vi "API Handle Value Change - Add to Owner.vi"(8 "Error In":errorcluster, 11 "Add to Owner New Value":bool) -> (0 "Error Out":errorcluster)   [LabVIEW 2022 SP3]
doc: "Enqueues a command."
uses:
  Command.ctl
panel:
  # "Development\ncontrols/indicators useful for development and testing, but which are not outputs of the VI"
  # "Input\nInputs to the VI"
  # "Output\nOutputs of the VI"
  # "Description\n\nBlank VI with error handling case. \n\nSummarize the use of this VI in this space."
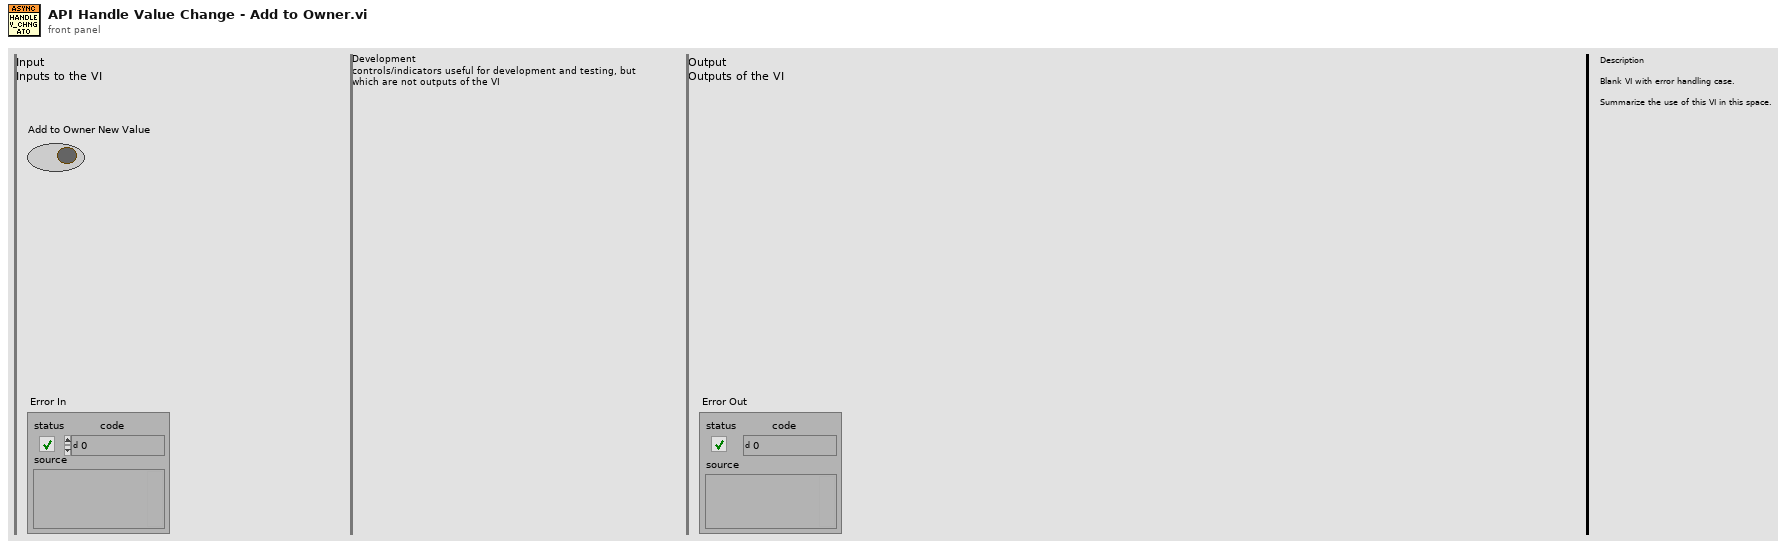
[diagram p1: front panel]
types:
  T1 = typedef "Command.ctl" = enum16{"Init Module", "Shutdown Module", "Local Error Handler", "Init Tickboxes", "Handle Value Change - Add to Project", "Handle Value Change - Add to Owner", "Handle Value Change - Add to Virtual Folder"}
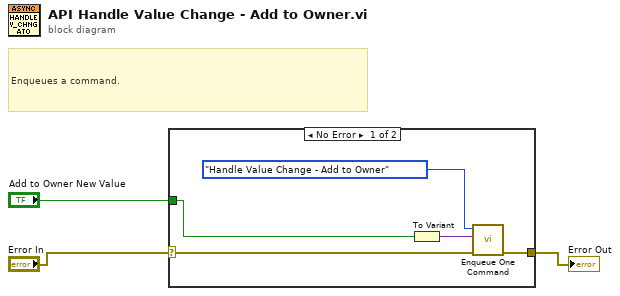
[diagram p0: block diagram]
diagram:
  # "Enqueues a command."
  n1 = case shown="No Error" "Error In" {
    selector: "Error In" -> [w7 w9]
    tunnel: [w6 w9] -> w2
    tunnel: "Add to Owner New Value" -> [w5 _]
    frame No Error {
      n2 = To Variant(anything=w5) -> (Variant=w4:variant)
      n3 = call "Enqueue One Command.vi"("error in (no error)"=w7, "Data"=w4, "Command"=Command."Handle Value Change - Add to Owner") -> ("error out"=w6:errorcluster)  [unwired: 8 in]
    }
    frame Error {
    }
  }
  "Error Out" <- w2
